vi "pbr-get-procs-names.vi"(8 "error in":errorcluster) -> (0 "error out":errorcluster, 3 "Array":string[](array[string]))   [LabVIEW 2024]
uses:
  controls/typePathSelector.ctl
  <vilib>/Utility/error.llb/Clear Errors.vi
  <vilib>/Utility/libraryn.llb/Create Directory Recursive.vi
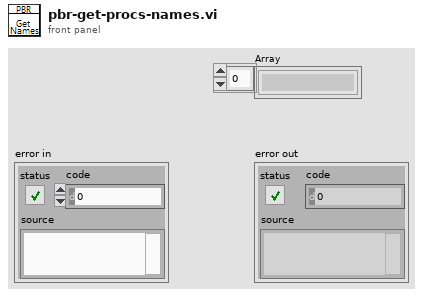
[diagram p1: front panel]
types:
  T1 = typedef "typePathSelector.ctl" = enum16{"DIR_PROCS", "DIR_CONFIG", "DIR_TEMPLATE", "DIR_IO_FILE", "DIR_RECORD", "DIR_LOG", "DIR_RUNTIME", "DIR_PRESET", "DIR_INI"}
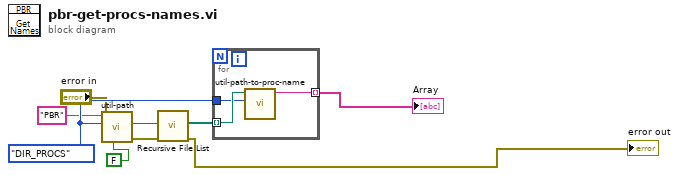
[diagram p0: block diagram]
diagram:
  w3 = typePathSelector."DIR_PROCS" ("Selected Folder (PROCS)")
  n1 = call "util-path.vi"("Create Folders?(F)"=FALSE, "error in"="error in", "Selected Folder (PROCS)"=w3, "append path (ie. folder\\filename.*)"="PBR" ("append path (ie. folder\\filename.*)")) -> ("error out"=w7:errorcluster, "SelectedPath"=w5:path)  [unwired: 3 in, 3 out]
  n2 = call <vilib>:"Recursive File List.vi"("error in (no error)"=w7, "Folder Path"=w5) -> ("error out"=→"error out":errorcluster, "All Files in Dir"=w8:path[])  [unwired: 5 in, 3 out]
  n3 = for {
    tunnel: [w10] -> w9 mode=indexing
    tunnel: w8 -> [w12] mode=indexing
    tunnel: w3 -> [w11]
    n4 = call "util-path-to-proc-name.vi"("location (DIR_PROCS)"=w11, "File path"=w12) -> ("String"=w10:string)  [unwired: 9 in]
  }
  "Array" <- w9
